vi "HXG2pidFGV_gainscheduling.vi"(0 "AirCool Cascade":T2={"PID gains"={"proportional gain (Kc)"=-1.15, "integral time (Ti, min)"=2.44, "derivative time (Td, min)"=0.0}, "output range"={"output high"=100.0, "output low"=10.0}} {"output range"."output low" format="%.2f"; "output range"."output high" format="%.2f"; "PID gains"."derivative time (Td, min)" format="%.3f"; "PID gains"."integral time (Ti, min)" format="%.3f"; "PID gains"."proportional gain (Kc)" format="%.3f"}, 1 "LiqHeat Cascade":T1={"PID gains"={"proportional gain (Kc)"=3.54, "integral time (Ti, min)"=46.25, "derivative time (Td, min)"=0.0}, "output range"={"output high"=100.0, "output low"=0.0}} {"output range"."output low" format="%.2f"; "output range"."output high" format="%.2f"; "PID gains"."derivative time (Td, min)" format="%.3f"; "PID gains"."integral time (Ti, min)" format="%.3f"; "PID gains"."proportional gain (Kc)" format="%.3f"}, 2 "PIDon-off In":T7, 3 "PID gains in":T3, 4 "PID Ref cluster":T6, 5 "error in (no error)":errorcluster, 6 "Reset PIDs":T4, 7 "PID Ctrls":T5, 10 "PIDfgvCtrl":T8) -> (9 "AirCool Cascade Out":T2={"PID gains"={"proportional gain (Kc)"=-1.15, "integral time (Ti, min)"=2.44, "derivative time (Td, min)"=0.0}, "output range"={"output high"=100.0, "output low"=10.0}} {"output range"."output low" format="%.2f"; "output range"."output high" format="%.2f"; "PID gains"."derivative time (Td, min)" format="%.3f"; "PID gains"."integral time (Ti, min)" format="%.3f"; "PID gains"."proportional gain (Kc)" format="%.3f"}, 11 "LiqHeat Cascade Out":T1={"PID gains"={"proportional gain (Kc)"=3.54, "integral time (Ti, min)"=46.25, "derivative time (Td, min)"=0.0}, "output range"={"output high"=100.0, "output low"=0.0}} {"output range"."output low" format="%.2f"; "output range"."output high" format="%.2f"; "PID gains"."derivative time (Td, min)" format="%.3f"; "PID gains"."integral time (Ti, min)" format="%.3f"; "PID gains"."proportional gain (Kc)" format="%.3f"}, 12 "PID Resets Out":T4, 13 "PID Ctrls Out":T5, 14 "Reset ON?":bool, 15 "PIDon-off":T7, 17 "PID Gains Out":T3, 18 "PID Refs Out":T6, 19 "error out":errorcluster)   [LabVIEW 2012]
uses:
  HXG2pid.ctl
  Controls/HXG2_PIDon-off.ctl
  CondensingVIs/PIDCtrl/HXG2_References.ctl
  Controls/HXG2_PIDctrlsOUT.ctl
  PID/HXG2_Horizontal Reset Control.ctl
  PID/HXG2_Horizontal PID Control.ctl
  Controls/HXG2_Aircool-Cascade.ctl
  Controls/HXG2_LiqHeat-Cascade.ctl
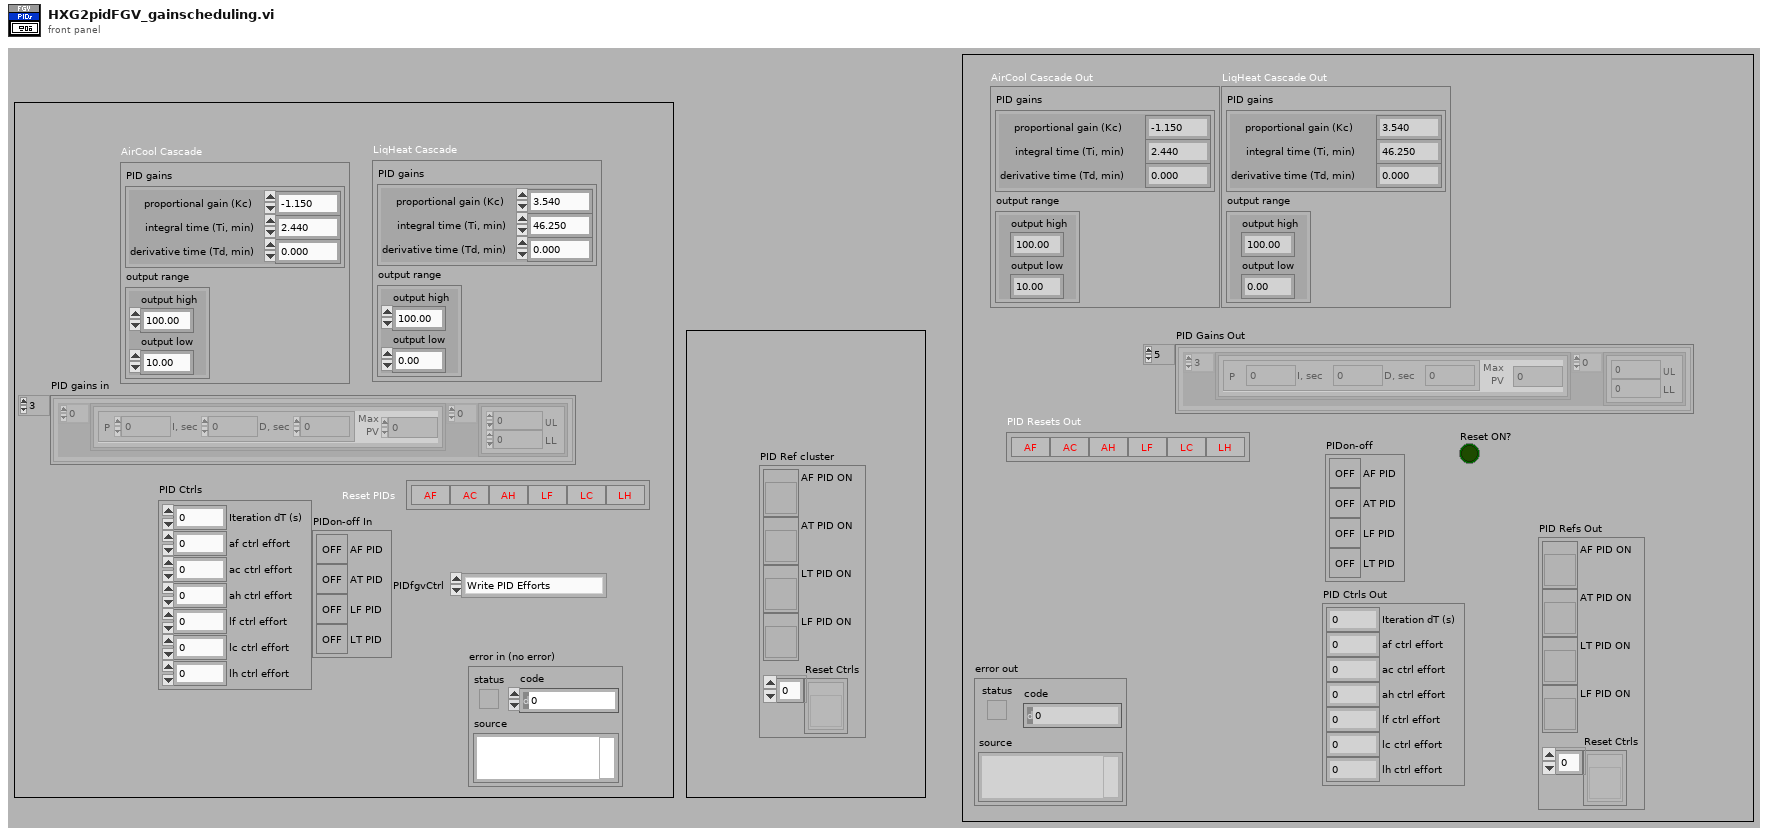
[diagram p1: front panel]
types:
  T1 = typedef "HXG2_LiqHeat-Cascade.ctl" = cluster{"PID gains":cluster{"proportional gain (Kc)":dbl, "integral time (Ti, min)":dbl, "derivative time (Td, min)":dbl}, "output range":cluster{"output high":dbl, "output low":dbl}}
  T2 = typedef "HXG2_Aircool-Cascade.ctl" = cluster{"PID gains":cluster{"proportional gain (Kc)":dbl, "integral time (Ti, min)":dbl, "derivative time (Td, min)":dbl}, "output range":cluster{"output high":dbl, "output low":dbl}}
  T3 = typedef "HXG2_Horizontal PID Control.ctl" = cluster{"GainsArray":cluster{"Gains 2":cluster{"P":dbl, "I, sec":dbl, "D, sec":dbl}, "Max\nPV":dbl}[], "UL-LL Array":cluster{"UL":dbl, "LL  ":dbl}[]}[]
  T4 = typedef "HXG2_Horizontal Reset Control.ctl" = cluster{"AF":bool, "AC":bool, "AH":bool, "LF":bool, "LC":bool, "LH":bool}
  T5 = typedef "HXG2_PIDctrlsOUT.ctl" = cluster{"Iteration dT (s)":dbl, "af ctrl effort":dbl, "ac ctrl effort":dbl, "ah ctrl effort":dbl, "lf ctrl effort":dbl, "lc ctrl effort":dbl, "lh ctrl effort":dbl}
  T6 = typedef "HXG2_References.ctl" = cluster{"AF PID ON":refnum<vi>, "AT PID ON":refnum<vi>, "LT PID ON":refnum<vi>, "LF PID ON":refnum<vi>, "Reset Ctrls":refnum<vi>[]}
  T7 = typedef "HXG2_PIDon-off.ctl" = cluster{"AF PID":bool, "AT PID":bool, "LF PID":bool, "LT PID":bool}
  T8 = typedef "HXG2pid.ctl" = enum16{"Write PID Efforts", "Write PID On-Off", "Pass", "Write PID Refs", "Write PID Gains", "Wrt PID Resets"}
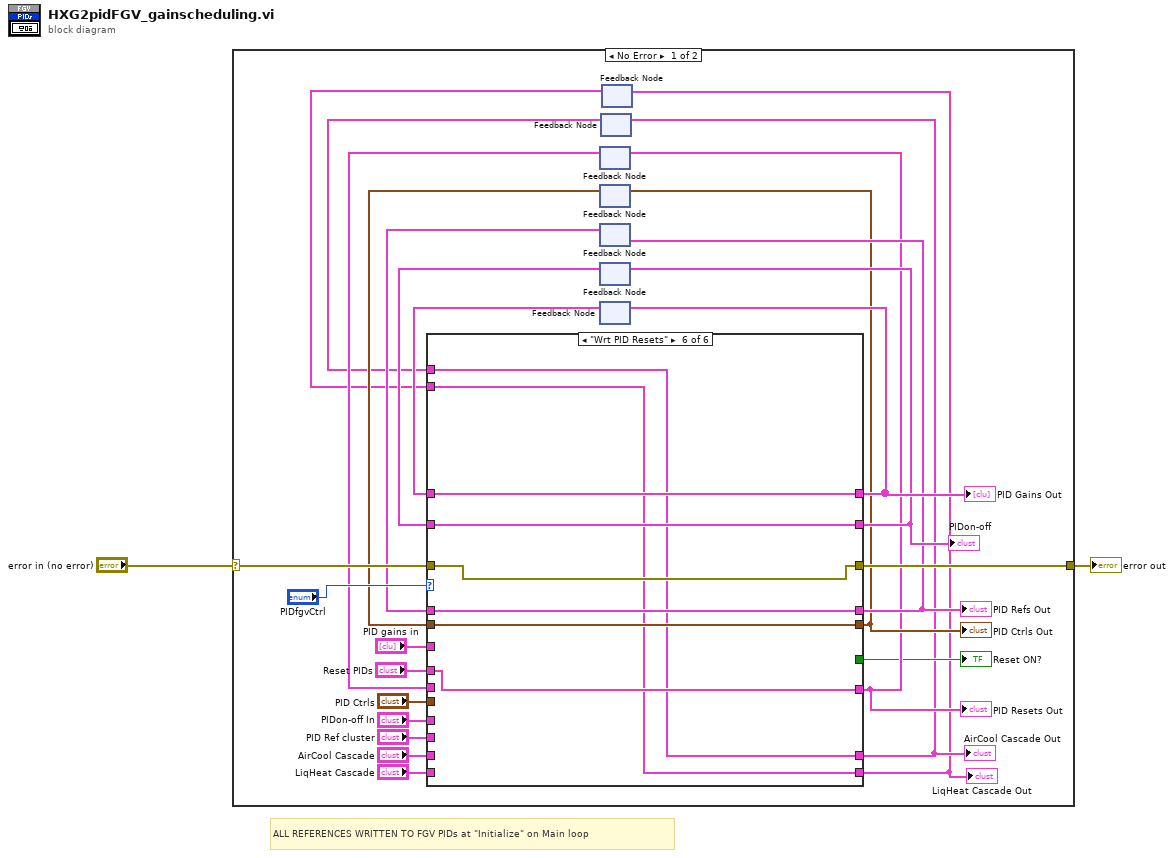
[diagram p0: block diagram]
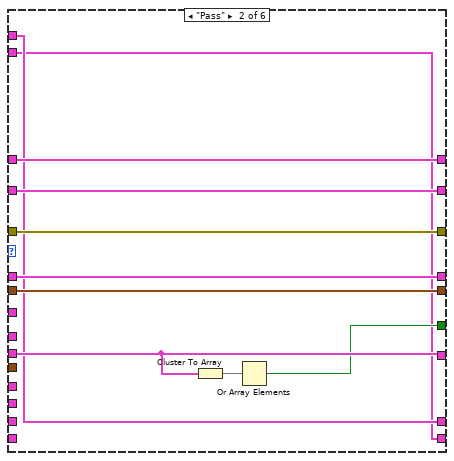
[diagram p3: hidden frame]
diagram:
  # "ALL REFERENCES WRITTEN TO FGV PIDs at \"Initialize\" on Main loop"
  n1 = case shown="No Error" "error in (no error)" {
    selector: "error in (no error)" -> [w27 w78]
    tunnel: [w26 w78] -> w1
    frame No Error {
      n2 = feedback #1() -> (w16:T4)  [unwired: 1 in]
      n3 = feedback #2() -> (w18:T5)  [unwired: 1 in]
      n4 = feedback #3() -> (w19:T6)  [unwired: 1 in]
      n5 = feedback #4() -> (w23:T7)  [unwired: 1 in]
      n6 = feedback #5() -> (w25:T3)  [unwired: 1 in]
      n7 = feedback #6() -> (w3:T2)  [unwired: 1 in]
      n8 = feedback #7() -> (w4:T1)  [unwired: 1 in]
      n9 = case shown="\"Wrt PID Resets\"" "PIDfgvCtrl" {
        tunnel: w27 -> [w35 w44 w52 w58 w66 w74]
        tunnel: [w35 w44 w52 w58 w66 w74] -> w26
        tunnel: [w32 w45 w53 w61 w64 w73] -> w22
        tunnel: w25 -> [w32 w45 w53 w61 _ w73]
        tunnel: [w34 w43 w48 w60 w69 w77] -> w21
        tunnel: w23 -> [w34 w43 _ w60 w69 w77]
        tunnel: [w33 w42 w50 w56 w68 w76] -> w20
        tunnel: w19 -> [w33 w42 w50 _ w68 w76]
        tunnel: [w30 w41 w51 w59 w67 w75] -> w17
        tunnel: w18 -> [_ w41 w51 w59 w67 w75]
        tunnel: [w31 w40 w49 w57 w65 w72] -> w14
        tunnel: w16 -> [w31 w40 w49 w57 _ _]
        tunnel: "Reset PIDs" -> [_ _ _ _ w65 w72]
        tunnel: [_ w38 _ _ _ _] -> w13
        tunnel: "PID gains in" -> [_ _ _ _ w64 _]
        tunnel: "PID Ctrls" -> [w30 _ _ _ _ _]
        tunnel: "PIDon-off In" -> [_ _ w48 _ _ _]
        tunnel: "PID Ref cluster" -> [_ _ _ w56 _ _]
        tunnel: "AirCool Cascade" -> [_ _ _ _ w63 _]
        tunnel: "LiqHeat Cascade" -> [_ _ _ _ w62 _]
        tunnel: [w29 w37 w47 w55 w63 w71] -> w6
        tunnel: [w28 w36 w46 w54 w62 w70] -> w5
        tunnel: w4 -> [w28 w36 w46 w54 _ w70]
        tunnel: w3 -> [w29 w37 w47 w55 _ w71]
        frame "Write PID Efforts" {
        }
        frame "Pass" {
          n10 = Cluster To Array(cluster=w40) -> (array=w39:bool[])
          n11 = Or Array Elements(Boolean array=w39) -> (logical OR=w38:bool)
        }
        frame "Write PID On-Off" {
        }
        frame "Write PID Refs" {
        }
        frame "Write PID Gains" {
        }
        frame "Wrt PID Resets" {
        }
      }
      "PIDon-off" <- w21
      "PID Refs Out" <- w20
      "PID Ctrls Out" <- w17
      "PID Resets Out" <- w14
      "PID Gains Out" <- w22
      "Reset ON?" <- w13
      "AirCool Cascade Out" <- w6
      "LiqHeat Cascade Out" <- w5
      n12 = feedback-in #1(w14) -> ()
      n13 = feedback-in #2(w17) -> ()
      n14 = feedback-in #3(w20) -> ()
      n15 = feedback-in #4(w21) -> ()
      n16 = feedback-in #5(w22) -> ()
      n17 = feedback-in #6(w6) -> ()
      n18 = feedback-in #7(w5) -> ()
    }
    frame Error {
    }
  }
  "error out" <- w1
